vi "Send image to image display controller - SubVI.vi"(0 "Image":T1, 1 "Window Title":string, 2 "Window Number":i32, 3 "error in":errorcluster, 4 "Image Type":T2 items=["Grayscale (U8)", "Grayscale (I16)", "Grayscale (SGL)", "Complex (CSG)", "RGB (U32)", "HSL (U32)", "RGB (U64)", "Grayscale (U16)"], 5 "Start display controller?":bool, 6 "Quit display controller?":bool) -> (7 "Image Out":T1, 10 "error out":errorcluster)   [LabVIEW 2014]
doc: "Uses a user event to send an image to Glimpse Image Display controller which is running in a separate thread, if both Start and Quit inputs are false.\n\nStart = TRUE launches the display controller as a separate thread; all other inputs are ignored.\n\nQuit = TRUE sends a message to the controller telling is to close the display windows and quit."
uses:
  <vilib>/vision/Image Controls.llb/IMAQ Image.ctl
  Glimpse-master/Glimpse core/Image to Display event.ctt
  Lambda Globals.vi
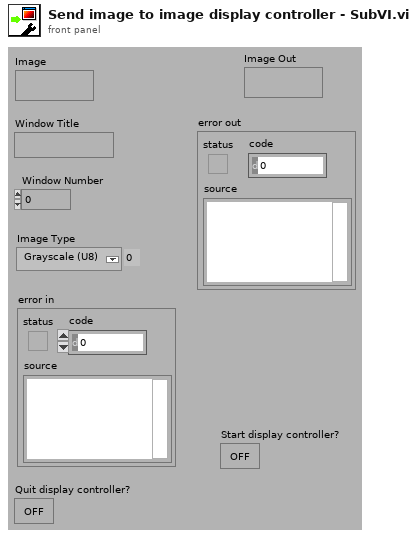
[diagram p1: front panel]
types:
  T1 = typedef "IMAQ Image.ctl" = refnum<image>
  T2 = typedef "Image Type" = u32
  T3 = typedef "Image to Display event.ctt" = cluster{"Image":T1, "Window Title":string, "Window Number":i32, "Image Type":T2, "Quit display controller?":bool}
  T4 = enum32{"Bad", "Idle", "Run top level", "Running"}
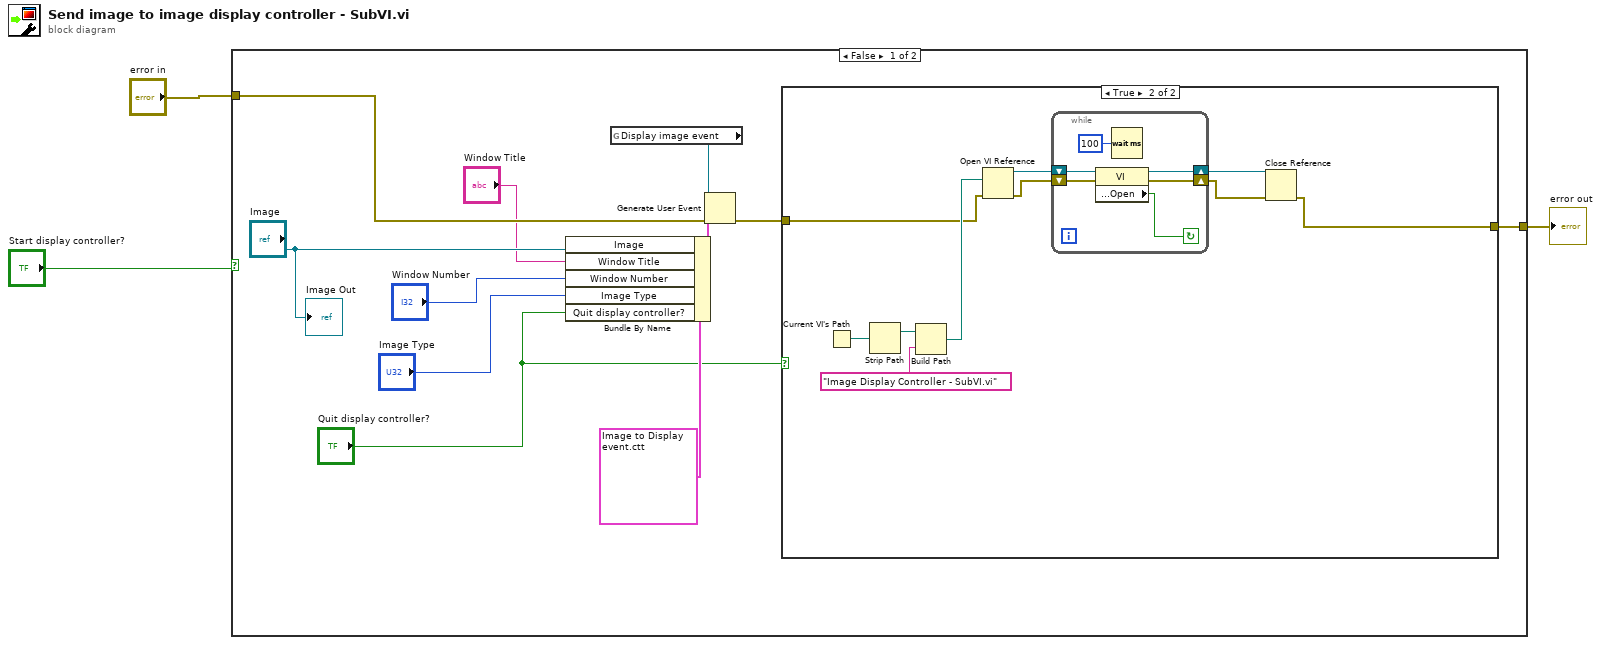
[diagram p0: block diagram]
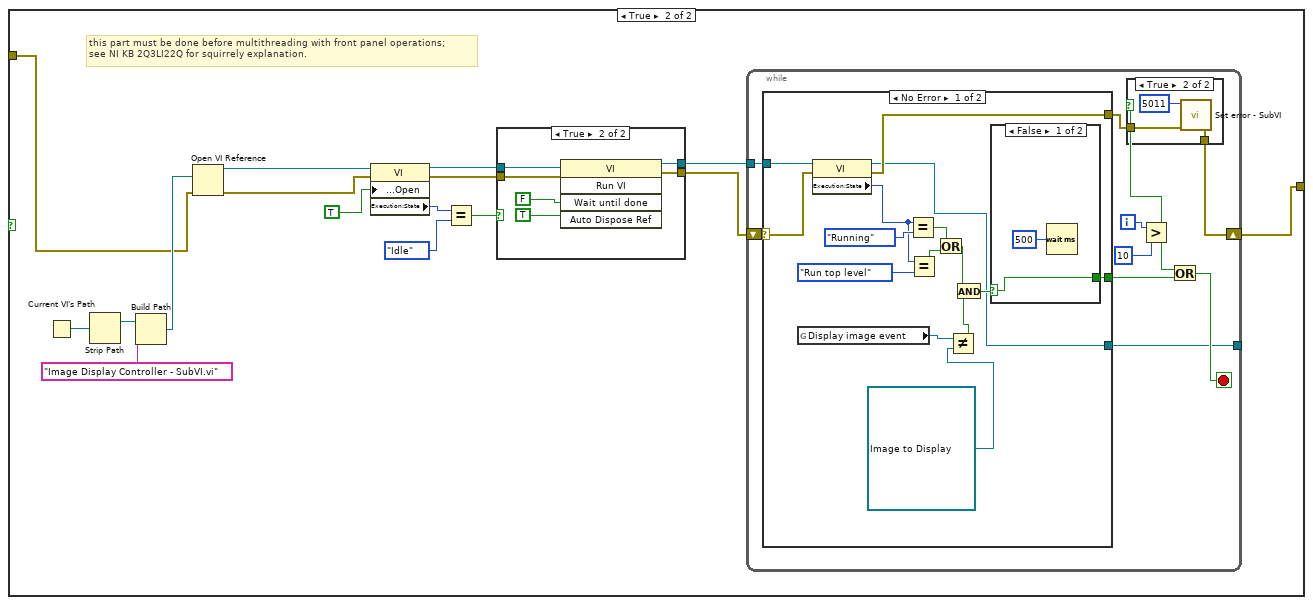
[diagram p3: hidden frame]
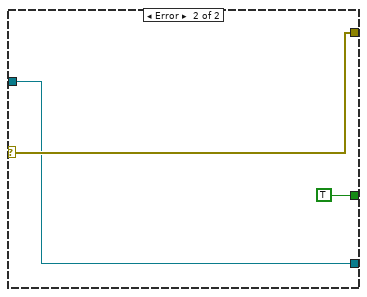
[diagram p7: hidden frame]
diagram:
  n1 = case shown="False" "Start display controller?" {
    tunnel: [w4 w42] -> w3
    tunnel: "error in" -> [w13 w43]
    frame False {
      n2 = Bundle By Name(cluster=T3 {"Image"=refnum, "Window Title"="", "Window Number"=0, "Image Type"=0, "Quit display controller?"=FALSE} ("event data"), "Image"="Image", "Window Title"="Window Title", "Window Number"="Window Number", "Image Type"="Image Type", "Quit display controller?"="Quit display controller?") -> (w10:T3)
      n3 = global read "Lambda Globals.vi" "Display image event"() -> (w12:refnum<user-event>)
      n4 = Generate User Event(user event=w12, event data cluster=w10, error in=w13) -> (error out=w6:errorcluster)  [unwired: 1 in, 1 out]
      n5 = case shown="True" "Quit display controller?" {
        tunnel: w6 -> [w15 w19]
        tunnel: [w15 w16] -> w4
        frame False {
        }
        frame True {
          n6 = Current VI's Path() -> (path=w21:path)
          n7 = Strip Path(path=w21) -> (stripped path=w20:path)  [unwired: 1 out]
          n8 = Build Path(base path=w20, name or relative path="Image Display Controller - SubVI.vi") -> (appended path=w23:path)
          n9 = Open VI Reference(vi path=w23, error in (no error)=w19) -> (vi reference=w25:refnum<vi>, error out=w24:errorcluster)  [unwired: 4 out]
          n10 = while {
            shift-right: [w27] -> w18
            shift-left: w25 -> [w31]
            shift-right: [w28] -> w17
            shift-left: w24 -> [w30]
            stop <- w29 continue-if-true
            n11 = property class="VI"(reference=w31, error in=w30) -> (reference out=w27:refnum<vi>, error out=w28:errorcluster, "Front Panel Window:Open"=w29:bool)
            n12 = Wait (ms)(milliseconds to wait=u32 100) -> ()  [unwired: 1 out]
          }
          n13 = Close Reference(reference=w18, error in (no error)=w17) -> (error out=w16:errorcluster)
        }
      }
      "Image Out" <- "Image"
    }
    frame True {
      # "this part must be done before multithreading with front panel operations;\nsee NI KB 2Q3LI22Q for squirrely explanation."
      n14 = Current VI's Path() -> (path=w45:path)
      n15 = Strip Path(path=w45) -> (stripped path=w44:path)  [unwired: 1 out]
      n16 = Build Path(base path=w44, name or relative path="Image Display Controller - SubVI.vi") -> (appended path=w47:path)
      n17 = Open VI Reference(vi path=w47, error in (no error)=w43) -> (vi reference=w38:refnum<vi>, error out=w37:errorcluster)  [unwired: 4 out]
      n18 = property class="VI"(reference=w38, error in=w37, "Front Panel Window:Open"=TRUE) -> (reference out=w39:refnum<vi>, error out=w36:errorcluster, "Execution:State"=w33:T4)
      n19 = Equal?(x=w33, y=T4."Idle" ("Execution:State")) -> (x = y?=w32:bool)
      n20 = case shown="True" w32 {
        tunnel: [w49 w54] -> w41
        tunnel: [w48 w53] -> w40
        tunnel: w39 -> [w49 w51]
        tunnel: w36 -> [w48 w50]
        frame False {
        }
        frame True {
          n21 = invoke class="VI" method="Run VI"(reference=w51, error in=w50, "Wait until done"=FALSE, "Auto Dispose Ref"=TRUE ("Wait until done")) -> (reference out=w54:refnum<vi>, error out=w53:errorcluster)  [unwired: 1 in, 3 out]
        }
      }
      n22 = while {
        tunnel: w41 -> [w65]
        shift-right: [w58] -> w42
        shift-left: w40 -> [w64]
        tunnel: [w56] -> _
        i -> [w63]
        stop <- w60 stop-if-true
        n23 = case shown="No Error" w64 {
          selector: w64 -> [w73 w89]
          tunnel: w65 -> [w76 w88]
          tunnel: [w74 TRUE] -> w61
          tunnel: [w72 w89] -> w59
          tunnel: [w71 w88] -> w56
          frame No Error {
            n24 = global read "Lambda Globals.vi" "Display image event"() -> (w82:refnum<user-event>)
            n25 = property class="VI"(reference=w76, error in=w73) -> (reference out=w71:refnum<vi>, error out=w72:errorcluster, "Execution:State"=w77:T4)
            n26 = Equal?(x=w77, y=T4."Running" ("Execution:State")) -> (x = y?=w81:bool)
            n27 = Equal?(x=w77, y=T4."Run top level" ("Execution:State")) -> (x = y?=w80:bool)
            n28 = Or(x=w81, y=w80) -> (x .or. y?=w83:bool)
            n29 = Not Equal?(x=w82, y=refnum<user-event> refnum ("Display image event")) -> (x != y?=w84:bool)
            n30 = And(x=w83, y=w84) -> (x .and. y?=w75:bool)
            n31 = case shown="False" w75 {
              selector: w75 -> [w85 w87]
              tunnel: [w85 w87] -> w74
              frame False {
                n32 = Wait (ms)(milliseconds to wait=u32 500) -> ()  [unwired: 1 out]
              }
              frame True {
              }
            }
          }
          frame Error {
          }
        }
        n33 = Greater?(x=w63, y=10) -> (0:w57:bool)
        n34 = case shown="True" w57 {
          tunnel: w59 -> [w66 w68]
          tunnel: [w66 w67] -> w58
          frame False {
          }
          frame True {
            n35 = call "Set error - SubVI.vi"("code"=5011, "error in"=w68) -> ("error out"=w67:errorcluster)  [unwired: 6 in]
          }
        }
        n36 = Or(x=w57, y=w61) -> (x .or. y?=w60:bool)
      }
    }
  }
  "error out" <- w3
